vi "DSF.Engine.Interface.Builder.Read.Response.vi"(8 "error in (no error)":errorcluster, 9 "timeout in ms (0)":i32 format="%d ms", 11 "Builder Interface in":refnum<class "DSF.Engine.Interface.Builder.lvclass">) -> (0 "error out":errorcluster, 1 "empty?":bool, 2 "response":T1, 3 "Builder Interface out":refnum<class "DSF.Engine.Interface.Builder.lvclass">, 4 "# elements":u32)   [LabVIEW 2016, in "DSF.Engine.lvlib" / "DSF.Engine.Interface.Builder.lvclass"]
uses:
  DSF.Engine.Interface.Builder.lvclass
  C:/Git/Sourcetree/DSF/Source/Engine/Classes/Interface/DSF.Engine.Interface.lvclass
  DSF.Engine.Interface.Builder.Response Data.ctl
  DSF.Engine.Interface.Builder.Response.ctl
  DSF.Engine.Interface.lvclass/DSF.Engine.Interface.ctl
  DSF.Engine.Interface.lvclass
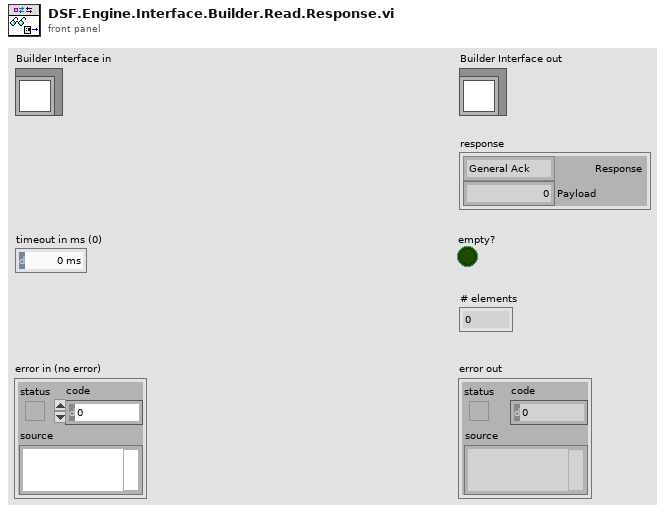
[diagram p1: front panel]
types:
  T1 = typedef "DSF.Engine.lvlib/DSF.Engine.Interface.Builder.lvclass/DSF.Engine.Interface.Builder.Response Data.ctl" = cluster{"Response":T2, "Payload":u64}
  T2 = typedef "DSF.Engine.lvlib/DSF.Engine.Interface.Builder.lvclass/DSF.Engine.Interface.Builder.Response.ctl" = enum8{"General Ack", "Shutdown Ack"}
  T3 = typedef "DSF.Engine.lvlib/DSF.Engine.Interface.lvclass/DSF.Engine.Interface.RT FIFO Ref.ctl" = refnum<k33>
  T4 = typedef "DSF.Engine.lvlib/DSF.Engine.Interface.lvclass/DSF.Engine.Interface.RT FIFO Data.ctl" = cluster{"Command":u8, "Payload":u64}
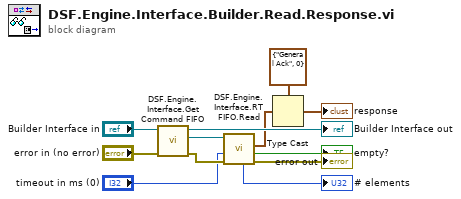
[diagram p0: block diagram]
diagram:
  n1 = call "DSF.Engine.Interface.Get Command FIFO.vi"("error in (no error)"="error in (no error)", "Interface in"="Builder Interface in") -> ("error out"=w11:errorcluster, "Command FIFO"=w12:T3, "Interface out"=→"Builder Interface out":refnum<class "DSF.Engine.Interface.Builder.lvclass">)  [unwired: 7 in]
  n2 = call "DSF.Engine.Interface.RT FIFO.Read.vi"("error in (no error)"=w11, "timeout in ms (0)"="timeout in ms (0)", "RT FIFO in"=w12) -> ("error out"=→"error out":errorcluster, "empty?"=→"empty?":bool, "element out"=w1:T4, "# elements"=→"# elements":u32)  [unwired: 4 in, 1 out]
  n3 = Type Cast(type=T1 {"Response"=enum."General Ack", "Payload"=0} ("Plugin Response"), x=w1) -> (*(type *) &x=→"response":T1)
